vi "ke37xx Digital I-O.vi"(0 "VISA Resource Name":refnum<visa-resource-name>, 5 "Action":T1(ring), 7 "Bit Number":u8=1 min=1 max=14 step=1, 9 "Bit Value To Write":u8=1 max=1 step=1, 11 "error in (no error)":errorcluster, 12 "Port Value To Write":u16=1 max=16383 step=1 format="%x", 13 "Mask":u16=1 max=16383 step=1 format="%x") -> (4 "VISA Resource Name Out":refnum<visa-resource-name>, 8 "Bit Value Read":u8 max=1 step=1, 10 "Port Value Read":u16 max=16383 step=1 format="%x", 15 "error out":errorcluster)   [LabVIEW 2009, in "Keithley 3700 Series.lvlib"]
doc: "This VI allows you to read from and write to the digital I/O port."
uses:
  <instrlib>/Keithley 3706/Keithley 3700 Series.lvlib
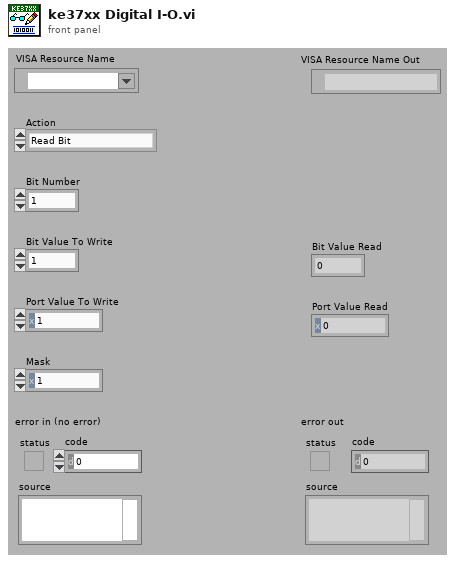
[diagram p1: front panel]
types:
  T1 = enum16{"Read Bit", "Read Port", "Write Bit", "Write Port", "Write Protect Mask"}
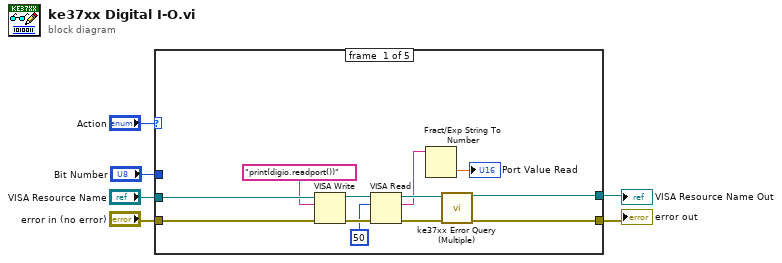
[diagram p0: block diagram]
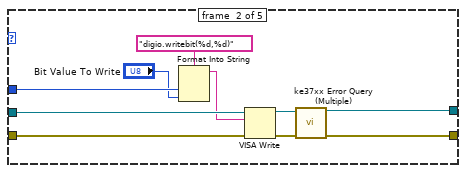
[diagram p2: hidden frame]
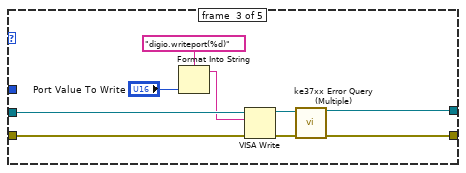
[diagram p3: hidden frame]
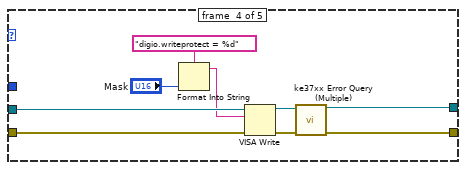
[diagram p4: hidden frame]
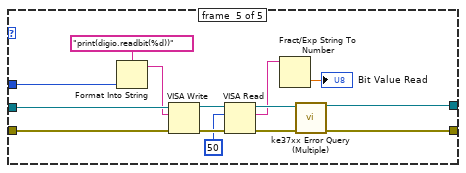
[diagram p5: hidden frame]
diagram:
  n1 = case shown="\"Write Protect Mask\"" "Action" {
    tunnel: "VISA Resource Name" -> [w18 w28 w37 w46 w60]
    tunnel: "error in (no error)" -> [w17 w27 w36 w45 w59]
    tunnel: [w16 w26 w35 w44 w58] -> w4
    tunnel: [w15 w25 w34 w43 w57] -> w3
    tunnel: "Bit Number" -> [_ w20 _ _ w47]
    frame #0 {
      n2 = VISA Write(VISA resource name=w18, write buffer="print(digio.readport())", error in (no error)=w17) -> (VISA resource name out=w14:refnum<visa-resource-name>, error out=w13:errorcluster)  [unwired: 1 out]
      n3 = VISA Read(VISA resource name=w14, byte count=u32 50, error in (no error)=w13) -> (VISA resource name out=w11:refnum<visa-resource-name>, read buffer=w9:string, error out=w12:errorcluster)  [unwired: 1 out]
      n4 = Fract/Exp String To Number(string=w9) -> (number=→"Port Value Read":dbl)  [unwired: 4 out]
      n5 = call <instrlib>:"ke37xx Error Query (Multiple).vi"("VISA resource name"=w11, "error in (no error)"=w12) -> ("VISA resource name out"=w16:refnum<visa-resource-name>, "error out"=w15:errorcluster)  [unwired: 12 out]
    }
    frame #1 {
      n6 = Format Into String(format string="digio.writebit(%d,%d)" ("write buffer"), w20, "Bit Value To Write") -> (resulting string=w21:string)  [unwired: 2 in, 1 out]
      n7 = VISA Write(VISA resource name=w28, write buffer=w21, error in (no error)=w27) -> (VISA resource name out=w24:refnum<visa-resource-name>, error out=w23:errorcluster)  [unwired: 1 out]
      n8 = call <instrlib>:"ke37xx Error Query (Multiple).vi"("VISA resource name"=w24, "error in (no error)"=w23) -> ("VISA resource name out"=w26:refnum<visa-resource-name>, "error out"=w25:errorcluster)  [unwired: 12 out]
    }
    frame #2 {
      n9 = Format Into String(format string="digio.writeport(%d)" ("write buffer"), "Port Value To Write") -> (resulting string=w30:string)  [unwired: 2 in, 1 out]
      n10 = VISA Write(VISA resource name=w37, write buffer=w30, error in (no error)=w36) -> (VISA resource name out=w33:refnum<visa-resource-name>, error out=w32:errorcluster)  [unwired: 1 out]
      n11 = call <instrlib>:"ke37xx Error Query (Multiple).vi"("VISA resource name"=w33, "error in (no error)"=w32) -> ("VISA resource name out"=w35:refnum<visa-resource-name>, "error out"=w34:errorcluster)  [unwired: 12 out]
    }
    frame #3 {
      n12 = Format Into String(format string="digio.writeprotect = %d" ("write buffer"), "Mask") -> (resulting string=w39:string)  [unwired: 2 in, 1 out]
      n13 = VISA Write(VISA resource name=w46, write buffer=w39, error in (no error)=w45) -> (VISA resource name out=w42:refnum<visa-resource-name>, error out=w41:errorcluster)  [unwired: 1 out]
      n14 = call <instrlib>:"ke37xx Error Query (Multiple).vi"("VISA resource name"=w42, "error in (no error)"=w41) -> ("VISA resource name out"=w44:refnum<visa-resource-name>, "error out"=w43:errorcluster)  [unwired: 12 out]
    }
    frame #4 {
      n15 = Format Into String(format string="print(digio.readbit(%d))" ("write buffer"), w47) -> (resulting string=w48:string)  [unwired: 2 in, 1 out]
      n16 = VISA Write(VISA resource name=w60, write buffer=w48, error in (no error)=w59) -> (VISA resource name out=w56:refnum<visa-resource-name>, error out=w55:errorcluster)  [unwired: 1 out]
      n17 = VISA Read(VISA resource name=w56, byte count=u32 50, error in (no error)=w55) -> (VISA resource name out=w53:refnum<visa-resource-name>, read buffer=w51:string, error out=w54:errorcluster)  [unwired: 1 out]
      n18 = Fract/Exp String To Number(string=w51) -> (number=→"Bit Value Read":dbl)  [unwired: 4 out]
      n19 = call <instrlib>:"ke37xx Error Query (Multiple).vi"("VISA resource name"=w53, "error in (no error)"=w54) -> ("VISA resource name out"=w58:refnum<visa-resource-name>, "error out"=w57:errorcluster)  [unwired: 12 out]
    }
  }
  "VISA Resource Name Out" <- w4
  "error out" <- w3
